vi "algo.runHostToFpgaTests.vi"() -> (3 "All Passed?":bool)   [LabVIEW 2022 SP3]
panel:
  out "Results":cluster{"Test Name":string, "Passed?":bool}[](array[cluster])
  out "# of Passed Tests":i32
  out "Seconds":u32
  out "Minutes":u32
  out "# of Test Results":i32
  out "Get All Control\nValues Variant":T1(array[cluster])
  out "error out":errorcluster
  in  "error in":errorcluster
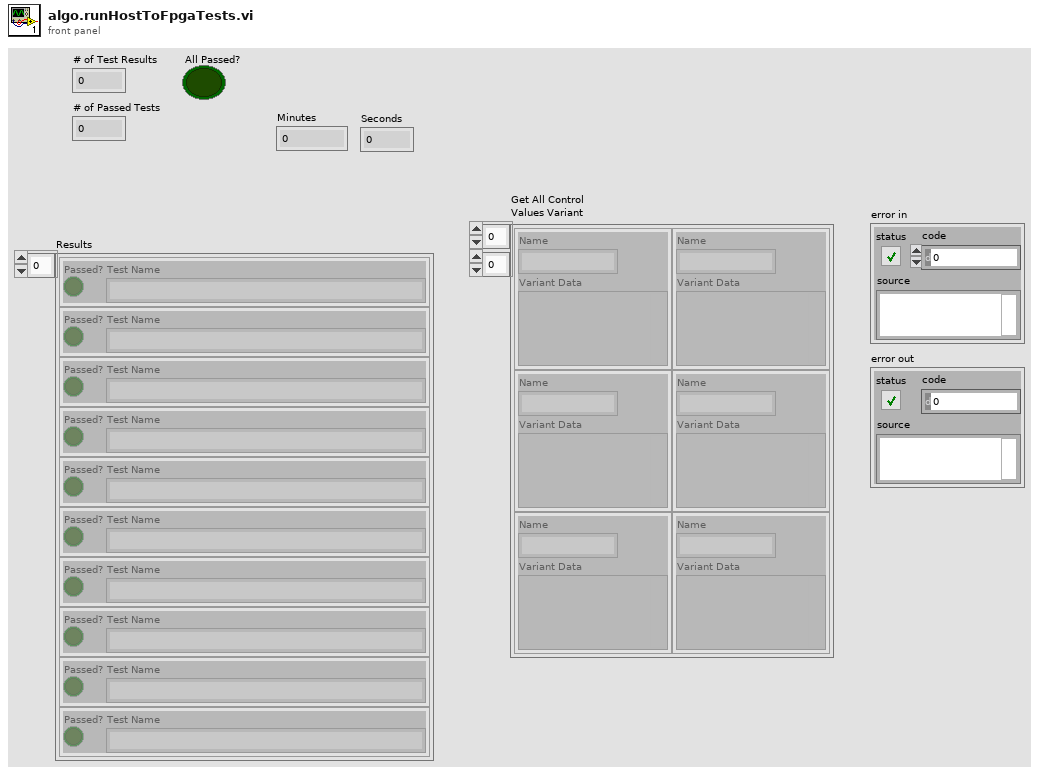
[diagram p1: front panel]
types:
  T1 = cluster{"Name":string, "Variant Data":variant}[][]
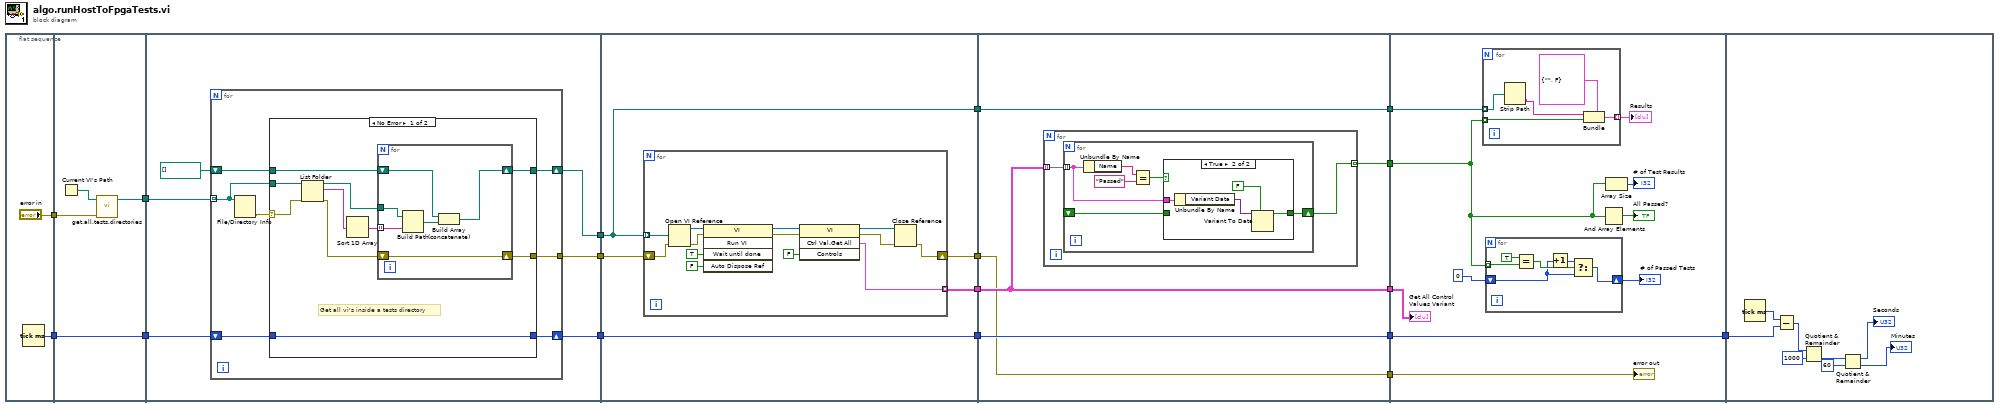
[diagram p0: block diagram]
diagram:
  n1 = flat-sequence {
    tunnel: [w19] -> w16
    tunnel: ["error in"] -> w9
    tunnel: [w23] -> w17
    tunnel: w16 -> [w23]
    tunnel: w9 -> [w20]
    tunnel: [w21] -> w8
    tunnel: w17 -> [w27]
    tunnel: [w29] -> w7
    tunnel: [w28] -> w3
    tunnel: w8 -> [w26]
    tunnel: [w24] -> w1
    tunnel: w7 -> [w57]
    tunnel: [w58] -> w6
    tunnel: [w59] -> w5
    tunnel: [w56] -> w4
    tunnel: w3 -> [w60]
    tunnel: [w60] -> w2
    tunnel: w1 -> [w56]
    tunnel: w6 -> [w74]
    tunnel: w5 -> [w75]
    tunnel: w4 -> [w78]
    tunnel: w2 -> [w77]
    tunnel: [w78] -> w15
    tunnel: [w77] -> w14
    tunnel: [w76] -> w13
    tunnel: [w75] -> w12
    tunnel: [w74] -> w11
    tunnel: w15 -> [w99]
    tunnel: w14 -> [w101]
    tunnel: w13 -> [w95]
    tunnel: w12 -> [w100]
    tunnel: w11 -> [w96]
    tunnel: [w101] -> w10
    tunnel: w10 -> [w119]
    frame #0 {
      n2 = Tick Count (ms)() -> (millisecond timer value=w19:u32)
    }
    frame #1 {
      n3 = Current VI's Path() -> (path=w22:path)
      n4 = call "get.all.tests.directories.vi"("error in"=w20, "Path.in"=w22) -> ("Test Directories"=w21:path[])  [unwired: 8 in, 1 out]
    }
    frame #2 {
      n5 = for {
        tunnel: [w36] -> w29
        shift-right: [w35] -> w28
        shift-left: w27 -> [w34]
        tunnel: w26 -> [w32] mode=indexing
        shift-right: [w30] -> w24
        shift-left: path[] [] -> [w31]
        n6 = File/Directory Info(path=w32) -> (error out=w33:errorcluster)  [unwired: 1 in, 6 out]
        n7 = case shown="No Error" w33 {
          selector: w33 -> [w45 w55]
          tunnel: w32 -> [w46 _]
          tunnel: [w42 w55] -> w36
          tunnel: w34 -> [w41 w54]
          tunnel: [w41 w54] -> w35
          tunnel: [w38 w53] -> w30
          tunnel: w31 -> [w37 w53]
          frame No Error {
            # "Get all vi's inside a tests directory"
            n8 = List Folder(path=w46, error in=w45) -> (path out=w44:path, filenames=w40:string[], error out=w43:errorcluster)  [unwired: 2 in, 1 out]
            n9 = Sort 1D Array(array=w40) -> (sorted array=w39:string[])
            n10 = for {
              tunnel: w44 -> [w52]
              shift-right: [w47] -> w42
              shift-left: w43 -> [w47]
              tunnel: w39 -> [w51] mode=indexing
              shift-right: [w49] -> w38
              shift-left: w37 -> [w48]
              n11 = Build Path(base path=w52, name or relative path=w51) -> (appended path=w50:path)
              n12 = Build Array (concatenate)(w48, w50) -> (w49:path[])
            }
          }
          frame Error {
          }
        }
      }
    }
    frame #3 {
      n13 = for {
        tunnel: [w64] -> w59 mode=indexing
        tunnel: w56 -> [w63] mode=indexing
        shift-right: [w62] -> w58
        shift-left: w57 -> [w61]
        n14 = Open VI Reference(vi path=w63, error in (no error)=w61) -> (vi reference=w73:refnum<vi>, error out=w72:errorcluster)  [unwired: 4 in]
        n15 = invoke class="VI" method="Run VI"(reference=w73, error in=w72, "Wait until done"=TRUE ("Wait Until Done"), "Auto Dispose Ref"=FALSE ("Auto Dispose Reference")) -> (reference out=w71:refnum<vi>, error out=w66:errorcluster)  [unwired: 1 in, 3 out]
        n16 = invoke class="VI" method="Ctrl Val.Get All"(reference=w71, error in=w66, "Controls"=FALSE) -> (reference out=w67:refnum<vi>, error out=w65:errorcluster, "Get All Control Values Variant"=w64:cluster{"Name":string, "Variant Data":variant}[])  [unwired: 1 in, 1 out]
        n17 = Close Reference(reference=w67, error in (no error)=w65) -> (error out=w62:errorcluster)
      }
    }
    frame #4 {
      n18 = for {
        tunnel: w75 -> [w80] mode=indexing
        tunnel: [w79] -> w76 mode=indexing
        n19 = for {
          tunnel: w80 -> [w83] mode=indexing
          shift-right: [w82] -> w79
          shift-left: _ -> [w81]
          n20 = Unbundle By Name(w83) -> ("Name"=w86:string)
          n21 = Equal?(x=w86, y="Passed") -> (x = y?=w84:bool)
          n22 = case shown="True" w84 {
            tunnel: w83 -> [_ w91]
            tunnel: [w87 w88] -> w82
            tunnel: w81 -> [w87 _]
            frame False {
            }
            frame True {
              n23 = Unbundle By Name(w91) -> ("Variant Data"=w90:variant)
              n24 = Variant To Data(type=FALSE, Variant=w90) -> (data=w88:bool)  [unwired: 1 in, 1 out]
            }
          }
        }
      }
    }
    frame #5 {
      n25 = for {
        tunnel: w99 -> [w109] mode=indexing
        tunnel: w95 -> [w112] mode=indexing
        tunnel: [w111] -> w92 mode=indexing
        n26 = Strip Path(path=w109) -> (name=w108:string)  [unwired: 1 out]
        n27 = Bundle(cluster=cluster{"Test Name":string, "Passed?":bool} {"Test Name"="", "Passed?"=FALSE}, "Test Name"=w108, "Passed?"=w112) -> (w111:cluster{"Test Name":string, "Passed?":bool})
      }
      "Results" <- w92
      n28 = for {
        tunnel: w95 -> [w107] mode=indexing
        shift-right: [w104] -> w93
        shift-left: 0 -> [w103]
        n29 = Equal?(x=TRUE, y=w107) -> (x = y?=w105:bool)
        n30 = Increment(x=w103) -> (x+1=w102:i32)
        n31 = Select(t=w102, s=w105, f=w103) -> (s? t:f=w104:i32)
      }
      "# of Passed Tests" <- w93
      n32 = And Array Elements(Boolean array=w95) -> (logical AND=→"All Passed?":bool)
      n33 = Array Size(array=w95) -> (size(s)=→"# of Test Results":i32)
      "Get All Control\nValues Variant" <- w100
      "error out" <- w96
    }
    frame #6 {
      n34 = Tick Count (ms)() -> (millisecond timer value=w120:u32)
      n35 = Subtract(x=w120, y=w119) -> (x-y=w118:u32)
      n36 = Quotient & Remainder(x=w118, y=u32 1000) -> (floor(x/y)=w116:u32)  [unwired: 1 out]
      n37 = Quotient & Remainder(x=w116, y=u32 60) -> (x-y*floor(x/y)=→"Seconds":u32, floor(x/y)=→"Minutes":u32)
    }
  }
